vi "Process-ARP.vi"(10 "Source Machine\nSettings":T1={"MAC Address"=[0, 1, 2, 3, 4, 5], "IP Address"=[10, 0, 1, 101]} {"MAC Address" format="%.0x"}, 11 "Frame (in)":u8[](array[numeric])=[0, 1, 8, 0, 6, 4, 0, 17, 0, 2, 201, 85, 8, 68, 10, 0, 1, 100, 0, 0, 0, 0, 0, 0, 10, 0, 1, 101, 0, 0, 0, 0, 0, 0, 0, 0, 0, 0, 0, 0, 0, 0, 0, 0, 0, 0, 124, 224, 175, 226, 255, 255, 255, 255] format="%02x") -> (1 "Response\nNeeded?":bool, 3 "ARP Response":u8[](array[numeric]) format="%02x")   [LabVIEW 2017]
uses:
  FPGANic/Source.Machine.Settings.ctl
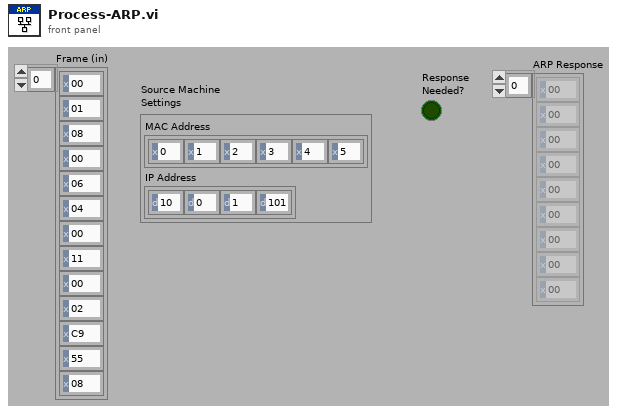
[diagram p1: front panel]
types:
  T1 = typedef "Source.Machine.Settings.ctl" = cluster{"MAC Address":u8[], "IP Address":u8[]}
  T2 = cluster{"HTYPE":u16, "PTYPE":u16, "HLEN":u8, "PLEN":u8, "OPER":u16}
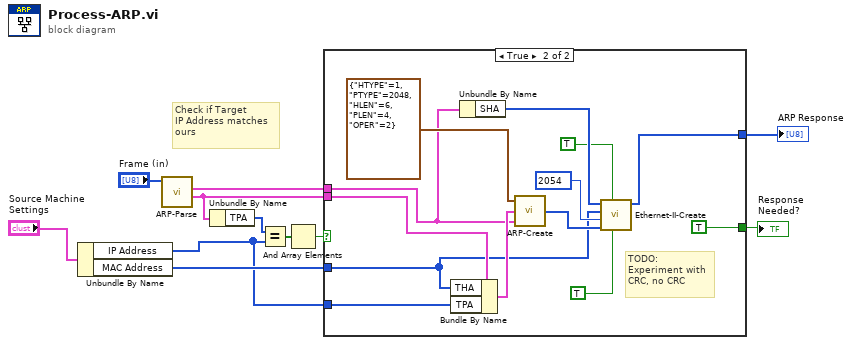
[diagram p0: block diagram]
diagram:
  # "Check if Target\nIP Address matches\nours"
  n1 = Unbundle By Name("Source Machine\nSettings") -> ("IP Address"=w1:u8[], "MAC Address"=w2:u8[])
  n2 = call "ARP-Parse.vi"("Frame (in)"="Frame (in)") -> ("Target"=w5:cluster{"THA":u8[], "TPA":u8[]}, "Sender"=w6:cluster{"SHA":u8[], "SPA":u8[]})  [unwired: 8 in, 1 out]
  n3 = Unbundle By Name(w5) -> ("TPA"=w9:u8[])
  n4 = Equal?(x=w9, y=w1) -> (x = y?=w8:bool[])
  n5 = And Array Elements(Boolean array=w8) -> (logical AND=w7:bool)
  n6 = case shown="True" w7 {
    tunnel: [_ TRUE] -> w11
    tunnel: w6 -> [_ w17]
    tunnel: w5 -> [_ w21]
    tunnel: w1 -> [_ w22]
    tunnel: w2 -> [_ w15]
    tunnel: [_ w14] -> w4
    frame False {
    }
    frame True {
      # "TODO:\nExperiment with\nCRC, no CRC"
      n7 = Bundle By Name(cluster=w21, "THA"=w15, "TPA"=w22) -> (w20:cluster{"THA":u8[], "TPA":u8[]})
      n8 = Unbundle By Name(w17) -> ("SHA"=w16:u8[])
      n9 = call "ARP-Create.vi"("Target"=w17, "Sender"=w20, "Header"=T2 {"HTYPE"=1, "PTYPE"=2048, "HLEN"=6, "PLEN"=4, "OPER"=2}) -> ("Arp Packet (out)"=w19:u8[])
      n10 = call "Ethernet-II-Create.vi"("Add CRC32?"=TRUE, "PadLen?"=TRUE, "Payload (in)"=w19, "EtherType"=u16 2054, "Source MAC"=w15, "Destination MAC"=w16) -> ("Ethernet Frame (out)"=w14:u8[])  [unwired: 5 in]
    }
  }
  "Response\nNeeded?" <- w11
  "ARP Response" <- w4
